vi "Merge Error.vi"(10 "Error":errorcluster, 11 "qqqqq in":refnum<class "qqqqq.lvclass">) -> (3 "qqqqq out":refnum<class "qqqqq.lvclass">)   [LabVIEW 2021, in "Providers.lvlib" / "qqqqq.lvlib" / "qqqqq.lvclass"]
uses:
  qqqqq.lvclass
  qqqqq.lvclass/qqqqq.ctl
  jettl/Queue/Queue.lvclass
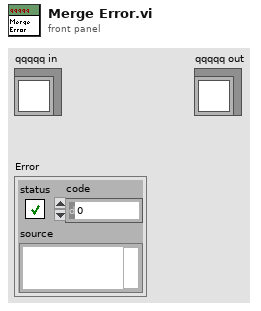
[diagram p1: front panel]
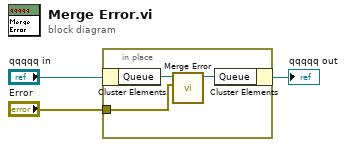
[diagram p0: block diagram]
diagram:
  n1 = in-place {
    in-place-border: "Error" -> [w6]
    n2 = in-place-cluster #1("qqqqq in") -> ("Queue"=w5:refnum<class "Queue.lvclass">)
    n3 = call-dynamic "Merge Error.vi"("Error"=w6, "Merge Error in"=w5) -> ("Merge Error out"=w4:refnum<class "Queue.lvclass">)  [unwired: 9 in]
    n4 = in-place-cluster #1("Queue"=w4) -> (→"qqqqq out":refnum<class "qqqqq.lvclass">)
  }
